vi "Main.vi"(8 "error in":errorcluster, 11 "Report in":refnum<class "Report.lvclass">) -> (0 "error out":errorcluster, 3 "Report out":refnum<class "Report.lvclass">)   [LabVIEW 2024, in "Report.lvclass"]
doc: "The <b>Queued Message Handler</b> of the Worker that owns this VI."
uses:
  Report.lvclass
  C:/Program Files (x86)/National Instruments/LabVIEW 2024/vi.lib/addons/_Workers/Library/Classes/Worker/Worker.lvclass
  Controller/rwr_Get Actual Data Reply.ctl
  Report.lvclass/Report.ctl
  rqp_Receive Log Interval.ctl
  Controller/Controller.lvclass
  <vilib>/Python/Open Venv Python Session.vi
  <vilib>/addons/_Workers/Library/Classes/Worker/Worker.lvclass
  <vilib>/addons/_Workers/Library/Classes/Message Queue/Message Queue.lvclass
  Initialization Data.ctl
panel:
  out "Report Entries":T1[](array[typedef]) {"Timestamp" format="%<%x %.3X>T"}
  out "Log Interval [ms]":i32=5000
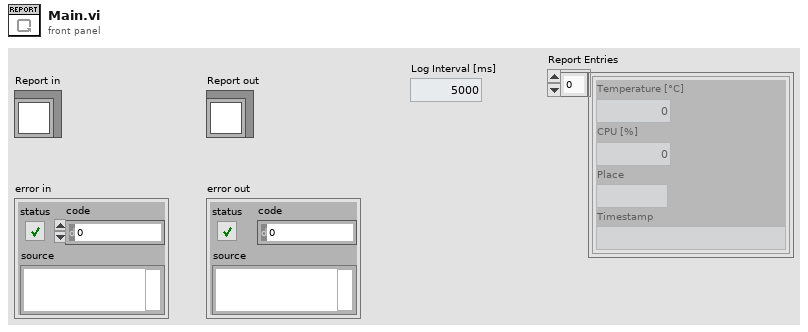
[diagram p1: front panel]
types:
  T1 = typedef "Controller.lvclass/rwr_Get Actual Data Reply.ctl" = cluster{"Temperature [°C]":dbl, "CPU [%]":dbl, "Place":string, "Timestamp":timestamp}
  T2 = typedef "Report.lvclass/Initialization Data.ctl" = cluster{"String":string, "Show Frontpanel":bool}
  T3 = enum32{"Invalid", "Standard", "Closed", "Hidden", "Minimized", "Maximized"}
  T4 = typedef "Report.lvclass/rqp_Receive Log Interval.ctl" = cluster{"Interval [ms]":i32}
  T5 = typedef "Workers.lvlib/Case Label.ctl" = string
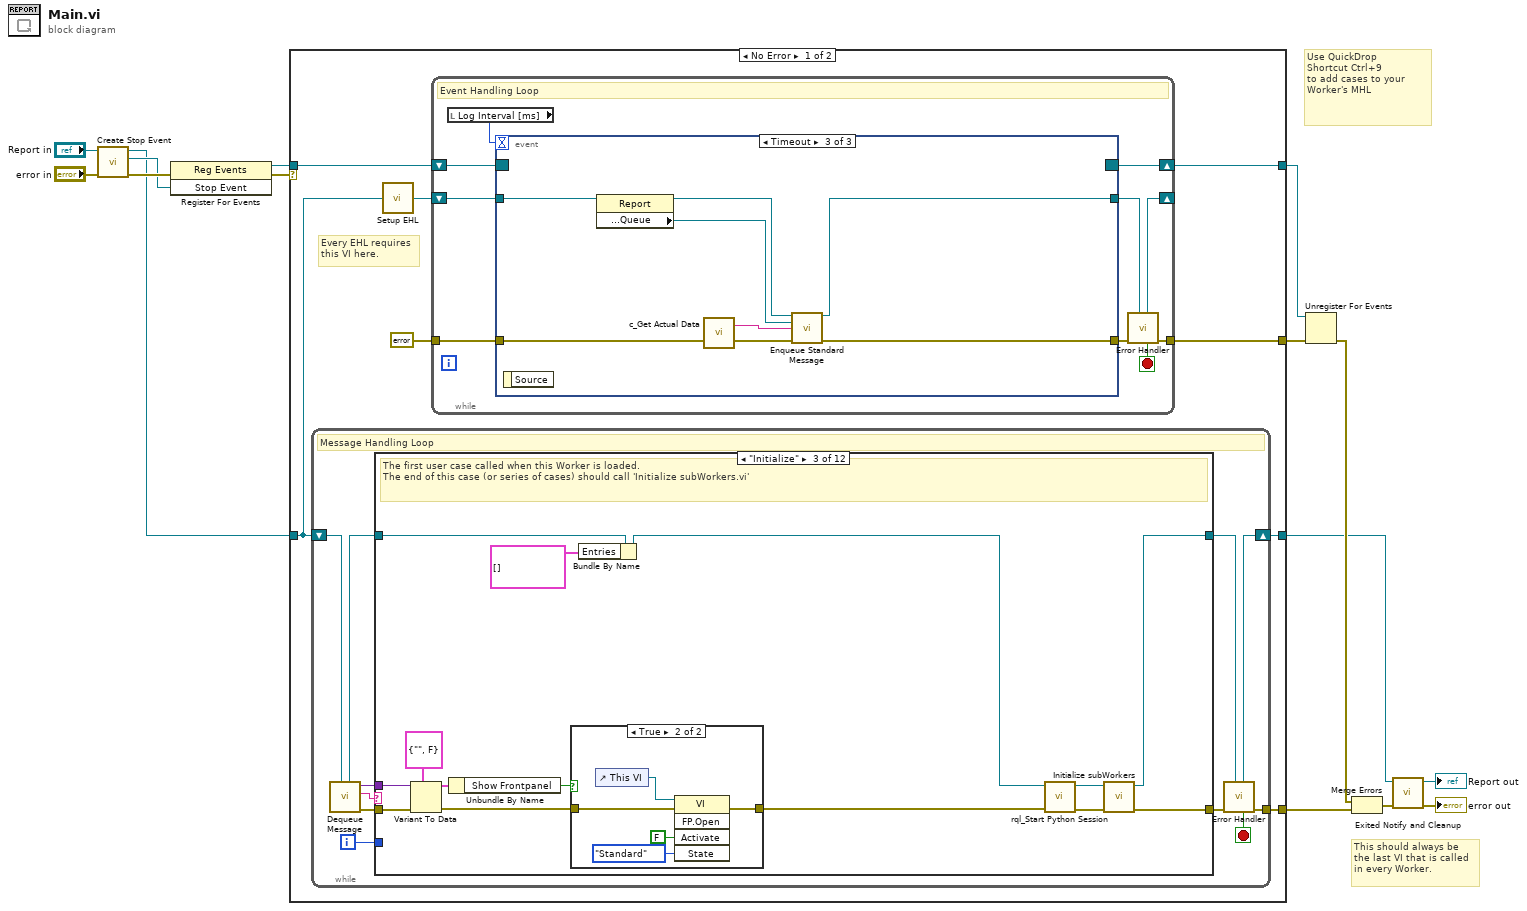
[diagram p0: block diagram]
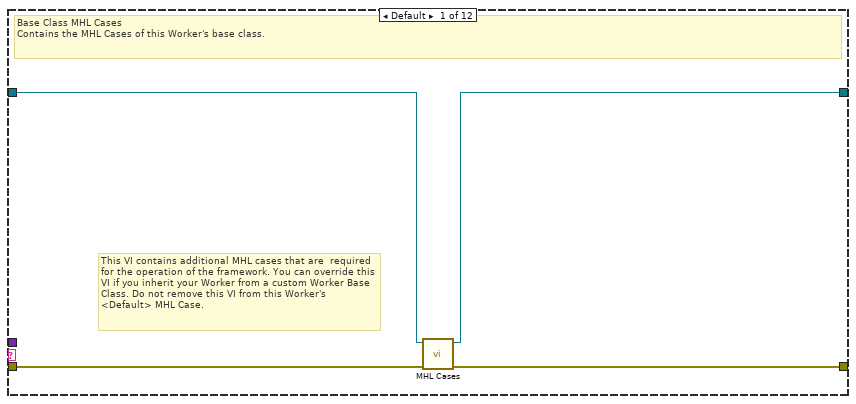
[diagram p2: hidden frame]
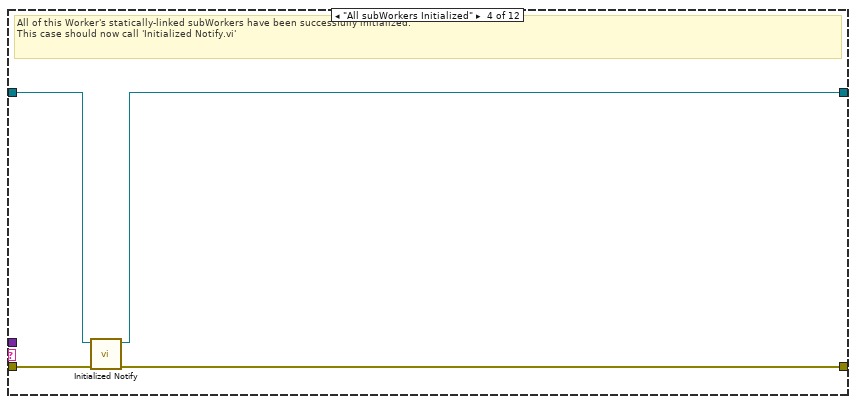
[diagram p5: hidden frame]
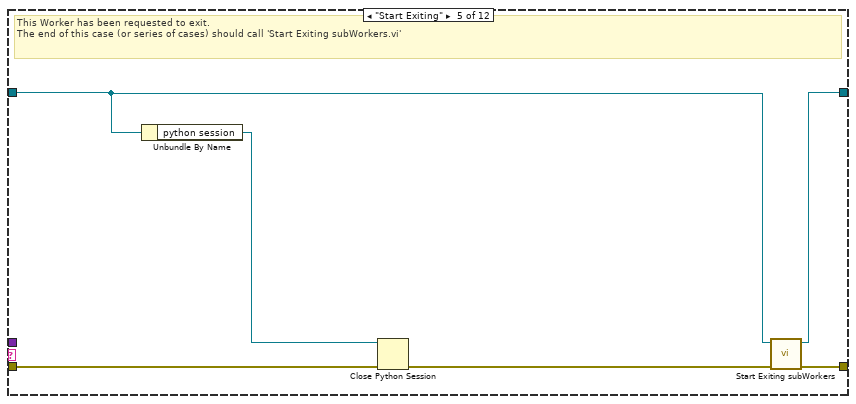
[diagram p6: hidden frame]
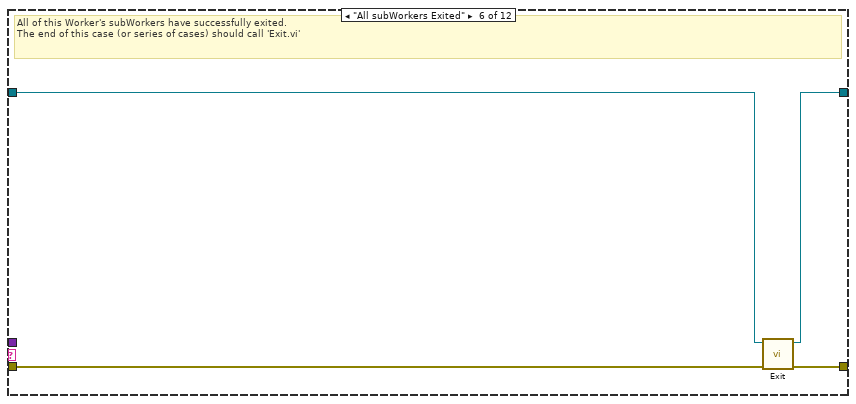
[diagram p7: hidden frame]
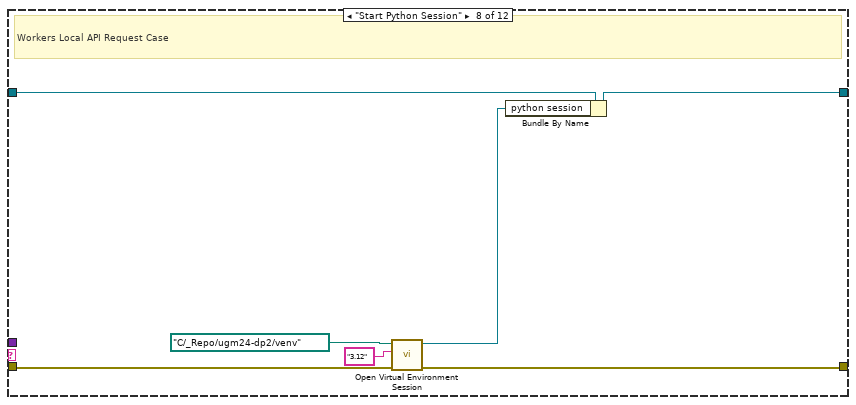
[diagram p9: hidden frame]
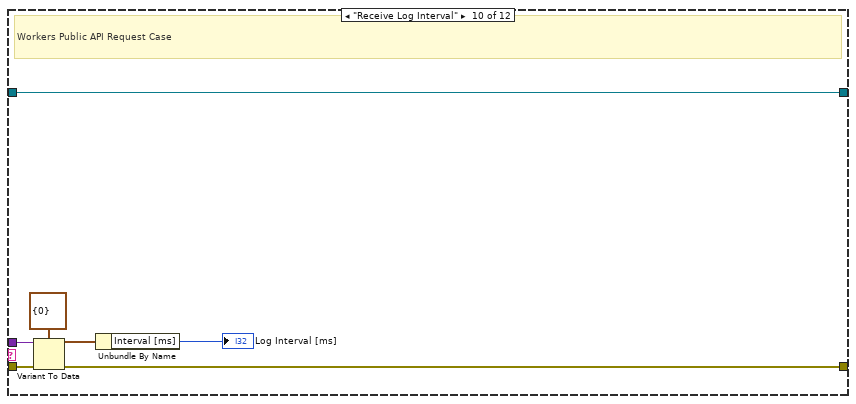
[diagram p11: hidden frame]
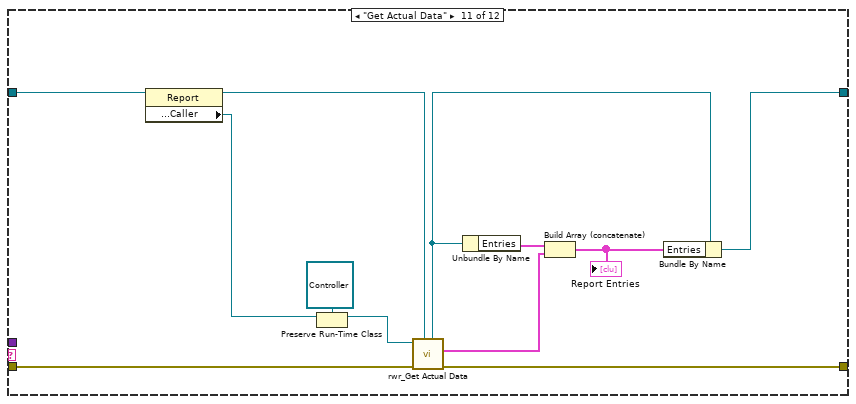
[diagram p12: hidden frame]
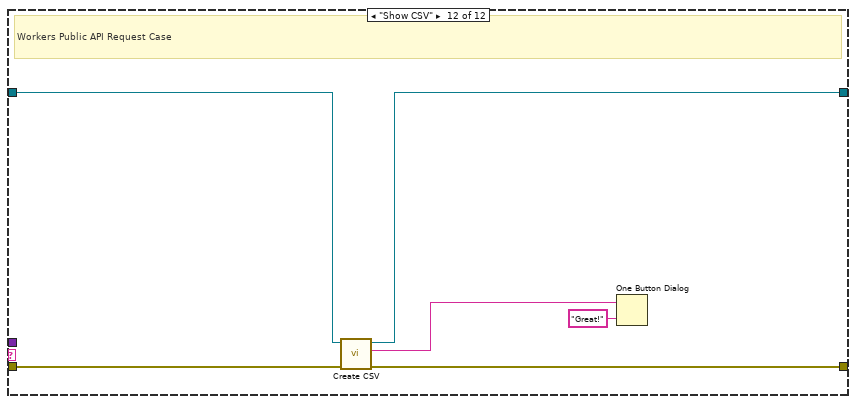
[diagram p13: hidden frame]
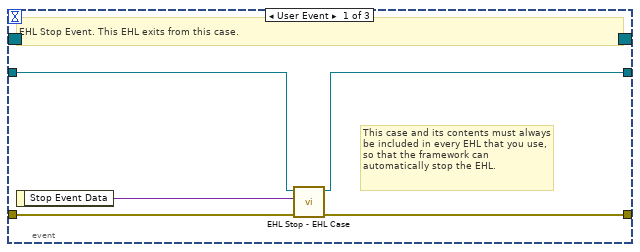
[diagram p14: hidden frame]
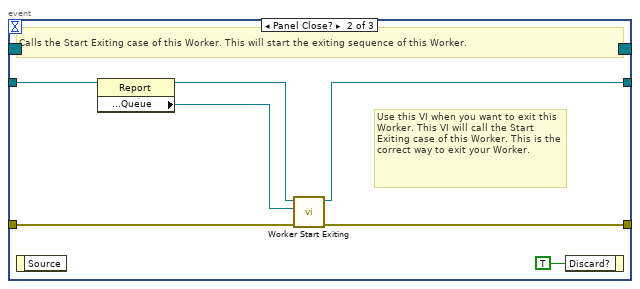
[diagram p15: hidden frame]
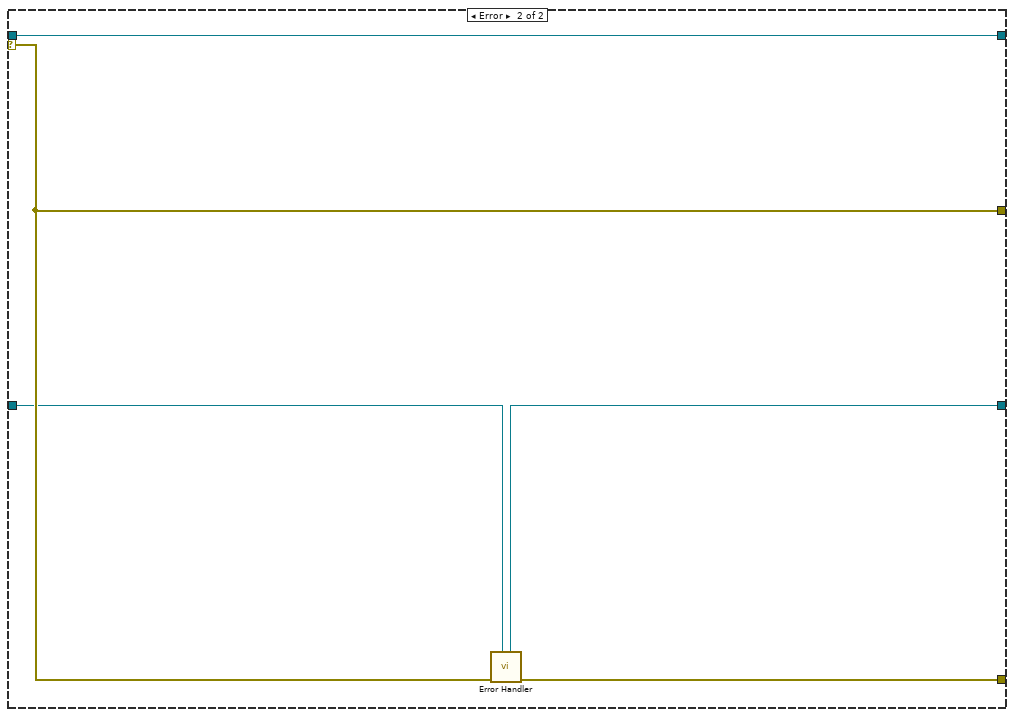
[diagram p16: hidden frame]
diagram:
  # "Use QuickDrop\nShortcut Ctrl+9\nto add cases to your\nWorker's MHL"
  # "This should always be the last VI that is called in every Worker."
  n1 = call-dynamic "Create Stop Event.vi"("error in"="error in", "Worker"="Report in") -> ("error out"=w10:errorcluster, "Stop Event"=w7:refnum<user-event>, "Worker out"=w4:refnum<class "Report.lvclass">)  [unwired: 7 in]
  n2 = register-events(error in=w10, w7) -> (reference out=w9:refnum<event-registration>, error out=w1:errorcluster)  [unwired: 1 in]
  n3 = case shown="No Error" w1 {
    tunnel: w4 -> [w18 w141]
    tunnel: [w16 w142] -> w8
    tunnel: w9 -> [w23 w143]
    tunnel: [w20 w144] -> w14
    tunnel: [w22 w143] -> w13
    tunnel: [w17 w140] -> w11
    selector: w1 -> [_ w144]
    frame No Error {
      # "Every EHL requires\nthis VI here."
      n4 = while {
        shift-right: [w32] -> w17
        shift-left: w18 -> [w34]
        tunnel: [w33] -> w16
        i -> [w25]
        stop <- w26 stop-if-true
        # "Message Handling Loop"
        n5 = call-dynamic "Dequeue Message.vi"("Worker"=w34) -> ("error out"=w31:errorcluster, "Case out"=w27:string, "Data out"=w24:variant, "Worker out"=w29:refnum<class "Report.lvclass">)  [unwired: 6 in, 1 out]
        n6 = case "Worker MHL Case Structure (DO NOT CHANGE LABEL NAME)" shown="\"Initialize\"" w27 {
          tunnel: w31 -> [w38 w39 w49 w62 w68 w74 w76 w80 w85 w91 w102 w110]
          tunnel: [w37 w39 w54 w61 w70 w73 w76 w79 w85 w90 w101 w109] -> w30
          tunnel: w29 -> [w36 w40 w50 w64 w67 w72 w75 w83 w84 w92 w104 w108]
          tunnel: [w35 w40 w53 w63 w69 w71 w75 w78 w84 w92 w94 w107] -> w28
          tunnel: w25 -> [_ _ _ _ _ _ _ _ _ _ _ _]
          tunnel: w24 -> [_ _ w46 _ _ _ _ _ _ w88 _ _]
          frame Default {
            # "This VI contains additional MHL cases that are  required for the operation of the framework. You can override this VI if you inherit your Worker from a custom Worker Base Class. Do not remove this VI from this Worker's <Default> MHL Case."
            # "Base Class MHL Cases\nContains the MHL Cases of this Worker's base class."
            n7 = call-dynamic "MHL Cases.vi"("error in"=w38, "Worker in"=w36) -> ("error out"=w37:errorcluster, "Worker out"=w35:refnum<class "Report.lvclass">)  [unwired: 8 in]
          }
          frame "------------ FRAMEWORK CASES -----------" {
            # "Start of Workers Framework Cases"
          }
          frame "Initialize" {
            # "The first user case called when this Worker is loaded.\nThe end of this case (or series of cases) should call 'Initialize subWorkers.vi'"
            n8 = Variant To Data(error in=w49, type=T2 {"String"="", "Show Frontpanel"=FALSE} ("Initialization Data"), Variant=w46) -> (data=w43:T2, error out=w44:errorcluster)
            n9 = Unbundle By Name(w43) -> ("Show Frontpanel"=w42:bool)
            n10 = case shown="True" w42 {
              tunnel: w44 -> [w55 w60]
              tunnel: [w55 w59] -> w41
              frame False {
              }
              frame True {
                n11 = control-ref of="This VI"() -> (w58:refnum<vi>)
                n12 = invoke class="VI" method="FP.Open"(reference=w58, error in=w60, "Activate"=FALSE ("Activate?"), "State"=T3."Standard") -> (error out=w59:errorcluster)  [unwired: 1 in, 4 out]
              }
            }
            n13 = Bundle By Name(cluster=w50, "Entries"=T1[] []) -> (w48:refnum<class "Report.lvclass">)
            n14 = call "rql_Start Python Session.vi"("error in"=w41, "CPU Percent in"=w48) -> ("error out"=w52:errorcluster, "dup CPU Percent out"=w51:refnum<class "Report.lvclass">)  [unwired: 8 in]
            n15 = call-dynamic "Initialize subWorkers.vi"("error in"=w52, "Worker"=w51) -> ("error out"=w54:errorcluster, "dup Worker out"=w53:refnum<class "Report.lvclass">)  [unwired: 8 in]
          }
          frame "All subWorkers Initialized" {
            # "All of this Worker's statically-linked subWorkers have been successfully initialized.\nThis case should now call 'Initialized Notify.vi'"
            n16 = call-dynamic "Initialized Notify.vi"("error in"=w62, "Worker"=w64) -> ("error out"=w61:errorcluster, "dup Worker out"=w63:refnum<class "Report.lvclass">)  [unwired: 8 in]
          }
          frame "Start Exiting" {
            # "This Worker has been requested to exit. \nThe end of this case (or series of cases) should call 'Start Exiting subWorkers.vi'"
            n17 = Unbundle By Name(w67) -> ("python session"=w65:refnum<k35>)
            n18 = Close Python Session(session in=w65, error in=w68) -> (11:w66:errorcluster)
            n19 = call-dynamic "Start Exiting subWorkers.vi"("error_in"=w66, "Worker"=w67) -> ("error out"=w70:errorcluster, "dup Worker out"=w69:refnum<class "Report.lvclass">)  [unwired: 8 in]
          }
          frame "All subWorkers Exited" {
            # "All of this Worker's subWorkers have successfully exited. \nThe end of this case (or series of cases) should call 'Exit.vi'"
            n20 = call-dynamic "Exit.vi"("error_in"=w74, "Worker"=w72) -> ("error out"=w73:errorcluster, "dup Worker out"=w71:refnum<class "Report.lvclass">)  [unwired: 8 in]
          }
          frame "------------- LOCAL API CASES -------------" {
            # "Start of Workers Local API Cases"
          }
          frame "Start Python Session" {
            # "Workers Local API Request Case"
            n21 = call-poly <vilib>:"Open Virtual Environment Session.vi"("error in (no error)"=w80, "Python version"="3.12", "Env path"=path "C:/_Repo/ugm24-dp2/venv") -> ("error out"=w79:errorcluster, "session out"=w77:refnum<k35>)  [unwired: 7 in]
            n22 = Bundle By Name(cluster=w83, "python session"=w77) -> (w78:refnum<class "Report.lvclass">)
          }
          frame "------------- PUBLIC API CASES -------------" {
            # "Start of Workers Public API Cases"
          }
          frame "Receive Log Interval" {
            # "Workers Public API Request Case"
            n23 = Variant To Data(error in=w91, type=T4 {"Interval [ms]"=0} ("Data"), Variant=w88) -> (data=w87:T4, error out=w90:errorcluster)
            n24 = Unbundle By Name(w87) -> ("Interval [ms]"=→"Log Interval [ms]":i32)
          }
          frame "Get Actual Data" {
            n25 = property class="Report"(reference=w104) -> (reference out=w100:refnum<class "Report.lvclass">, "Accessors:Read:Public API:Caller"=w103:refnum<class "Worker.lvclass">)  [unwired: 1 in, 1 out]
            n26 = Preserve Run-Time Class(object in=w103, 2:refnum<class "Controller.lvclass"> refnum ("Controller")) -> (object out=w99:refnum<class "Controller.lvclass">)  [unwired: 1 in, 1 out]
            n27 = call "rwr_Get Actual Data.vi"("Caller in"=w100, "error in"=w102, "Controller in"=w99) -> ("error out"=w101:errorcluster, "Reply Data out"=w95:T1, "dup Caller out"=w97:refnum<class "Report.lvclass">)  [unwired: 5 in, 1 out]
            n28 = Unbundle By Name(w97) -> ("Entries"=w96:T1[])
            n29 = Build Array (concatenate)(w96, w95) -> (w93:T1[])
            "Report Entries" <- w93
            n30 = Bundle By Name(cluster=w97, "Entries"=w93) -> (w94:refnum<class "Report.lvclass">)
          }
          frame "Show CSV" {
            # "Workers Public API Request Case"
            n31 = call "Create CSV.vi"("error in (no error)"=w110, "Report in"=w108) -> ("error out"=w109:errorcluster, "CSV"=w106:string, "Report out"=w107:refnum<class "Report.lvclass">)  [unwired: 7 in]
            n32 = One Button Dialog(message=w106, button name ("OK")="Great!") -> ()  [unwired: 1 out]
          }
        }
        n33 = call-dynamic "Error Handler.vi"("Worker"=w28, "error_in"=w30) -> ("error out"=w33:errorcluster, "Stop Loop"=w26:bool, "Worker out"=w32:refnum<class "Report.lvclass">)  [unwired: 7 in]
      }
      n34 = call-dynamic "Setup EHL.vi"("Worker"=w18) -> ("Worker out"=w19:refnum<class "Report.lvclass">)  [unwired: 14 in]
      n35 = while "Event Handling Loop" {
        shift-right: [w120] -> w22
        shift-left: w23 -> [w119]
        tunnel: [w115] -> w20
        tunnel: errorcluster {"status"=FALSE, "code"=0, "source"=""} ("error constant") -> [w117]
        shift-right: [w113] -> _
        shift-left: w19 -> [w118]
        stop <- w112 stop-if-true
        # "Event Handling Loop"
        n36 = local read "Log Interval [ms]"() -> (w111:i32)
        n37 = event shown="[2] Timeout" {
          selector: w119 -> [_ _ _]
          dyn-events: [_ _ _] -> w120
          timeout: w111 -> [_ _ _]
          tunnel: [w124 w131 w138] -> w116
          tunnel: w117 -> [w125 w130 w139]
          tunnel: w118 -> [w123 w129 w137]
          tunnel: [w122 w128 w136] -> w114
          event User Event {
            # "This case and its contents must always be included in every EHL that you use, so that the framework can automatically stop the EHL."
            # "EHL Stop Event. This EHL exits from this case."
            n38 = event-data() -> ("Stop Event Data"=w121:variant)  [unwired: 1 in]
            n39 = call-dynamic "EHL Stop - EHL Case.vi"("error in"=w125, "Stop Event Data"=w121, "Worker"=w123) -> ("error out"=w124:errorcluster, "Worker out"=w122:refnum<class "Report.lvclass">)  [unwired: 7 in]
          }
          event Panel Close? {
            # "Use this VI when you want to exit this Worker. This VI will call the Start Exiting case of this Worker. This is the correct way to exit your Worker."
            # "Calls the Start Exiting case of this Worker. This will start the exiting sequence of this Worker."
            n40 = event-data() -> ()  [unwired: 1 in, 1 out]
            n41 = property class="Report"(reference=w129) -> (reference out=w127:refnum<class "Report.lvclass">, "Accessors:Read:Public API:Queue"=w126:refnum<class "Message Queue.lvclass">)  [unwired: 1 in, 1 out]
            n42 = call-dynamic "Worker Start Exiting.vi"("error_in"=w130, "Message Queue"=w126, "Worker"=w127) -> ("error out"=w131:errorcluster, "dup Worker out"=w128:refnum<class "Report.lvclass">)  [unwired: 7 in]
            n43 = event-data("Discard?"=TRUE) -> ()  [unwired: 1 in, 1 out]
          }
          event Timeout {
            n44 = event-data() -> ()  [unwired: 1 in, 1 out]
            n45 = property class="Report"(reference=w137) -> (reference out=w134:refnum<class "Report.lvclass">, "Accessors:Read:Public API:Queue"=w133:refnum<class "Message Queue.lvclass">)  [unwired: 1 in, 1 out]
            n46 = call "c_Get Actual Data.vi"() -> ("Case Label"=w135:T5)  [unwired: 1 in]
            n47 = call-dynamic "Enqueue Standard Message.vi"("Worker"=w134, "Message Queue"=w133, "Case Label"=w135, "error in (no error)"=w139) -> ("dup Worker out"=w136:refnum<class "Report.lvclass">, "error out"=w138:errorcluster)  [unwired: 10 in]
          }
        }
        n48 = call-dynamic "Error Handler.vi"("Worker"=w114, "error_in"=w116) -> ("error out"=w115:errorcluster, "Stop Loop"=w112:bool, "Worker out"=w113:refnum<class "Report.lvclass">)  [unwired: 7 in]
      }
    }
    frame Error {
      n49 = call-dynamic "Error Handler.vi"("Worker"=w141, "error_in"=w144) -> ("error out"=w142:errorcluster, "Worker out"=w140:refnum<class "Report.lvclass">)  [unwired: 7 in, 1 out]
    }
  }
  n50 = Unregister For Events(event registration refnum=w13, error in=w14) -> (error out=w15:errorcluster)
  n51 = Merge Errors(w15, w8) -> (w12:errorcluster)
  n52 = call-dynamic "Exited Notify and Cleanup.vi"("error_in"=w12, "Worker"=w11) -> ("error out"=→"error out":errorcluster, "dup Worker out"=→"Report out":refnum<class "Report.lvclass">)  [unwired: 8 in]
